vi "test_LocationFGV_ReresolveLocationTwice_LocationResolvedTwice.vi"(8 "error in":errorcluster) -> (0 "error out":errorcluster, 2 "result":string, 3 "pass":bool)   [LabVIEW 2020, in "MeasurementServerTests.lvlib" / "Discovery Tests.lvlib"]
uses:
  Discovery Tests.lvlib
  Fake Service Location Generator Action.ctl
  Runtime/MeasurementLink Discovery V1/TypeDefs/Service Location FGV Action.ctl
  Runtime/MeasurementLink Discovery V1/MeasurementLink Discovery V1.lvlib
  Runtime/Generated/Measurement Plugin Discovery Client/RPC Messages/ni_measurementlink_discovery_v1_ResolveServiceRequest.ctl
  Runtime/Generated/Measurement Plugin Discovery Client/Measurement Plugin Discovery Client.lvlib
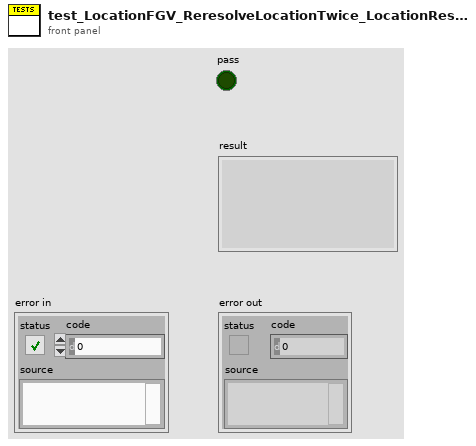
[diagram p1: front panel]
types:
  T1 = typedef "Measurement Plugin Discovery Client.lvlib/ni_measurementlink_discovery_v1_ResolveServiceRequest.ctl" = cluster{"provided_interface":string, "service_class":string}
  T2 = typedef "MeasurementLink Discovery V1.lvlib/Service Location FGV Action.ctl" = enum16{"Get Service Location", "Reresolve Service Location"}
  T3 = typedef "MeasurementServerTests.lvlib/Discovery Tests.lvlib/Fake Service Location Generator Action.ctl" = enum16{"Generate New Location", "Reset", "Error on Next Call"}
  T4 = typedef "Measurement Plugin Discovery Client.lvlib/ni_measurementlink_discovery_v1_ServiceLocation.ctl" = cluster{"location":string, "insecure_port":string, "ssl_authenticated_port":string}
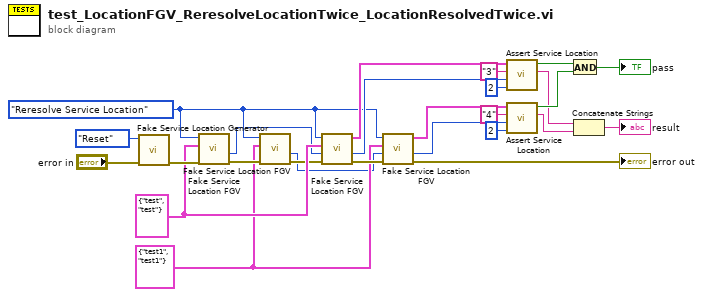
[diagram p0: block diagram]
diagram:
  w14 = T1 {"provided_interface"="test1", "service_class"="test1"} ("resolve service request")
  w23 = T1 {"provided_interface"="test", "service_class"="test"} ("resolve service request")
  w15 = Service_Location_FGV_Action."Reresolve Service Location" ("action")
  n1 = call "Fake Service Location Generator.vi"("error in"="error in", "action"=Fake_Service_Location_Generator_Action."Reset") -> ("error out"=w25:errorcluster)  [unwired: 8 in, 1 out]
  n2 = call "Fake Service Location FGV.vi"("error in"=w25, "resolve service request"=w23, "action"=w15) -> ("error out"=w18:errorcluster, "unique id out"=w2:u64)  [unwired: 6 in, 1 out]
  n3 = call "Fake Service Location FGV.vi"("error in"=w18, "resolve service request"=w14, "action"=w15) -> ("error out"=w17:errorcluster, "unique id out"=w1:u64)  [unwired: 6 in, 1 out]
  n4 = call "Fake Service Location FGV.vi"("error in"=w17, "unique id in"=w2, "resolve service request"=w23, "action"=w15) -> ("error out"=w16:errorcluster, "unique id out"=w20:u64, "service location"=w22:T4)  [unwired: 5 in]
  n5 = call "Fake Service Location FGV.vi"("error in"=w16, "unique id in"=w1, "resolve service request"=w14, "action"=w15) -> ("error out"=→"error out":errorcluster, "unique id out"=w9:u64, "service location"=w10:T4)  [unwired: 5 in]
  n6 = call "Assert Service Location.vi"("expected unique id"=u64 2, "actual unique id"=w20, "expected service location port"="3", "actual service location"=w22) -> ("result"=w5:string, "pass"=w19:bool)  [unwired: 6 in]
  n7 = call "Assert Service Location.vi"("expected unique id"=u64 2, "actual unique id"=w9, "expected service location port"="4", "actual service location"=w10) -> ("result"=w4:string, "pass"=w6:bool)  [unwired: 6 in]
  n8 = And(x=w19, y=w6) -> (x .and. y?=→"pass":bool)
  n9 = Concatenate Strings(w5, w4) -> (→"result":string)
